vi "sta_Correlation Coefficient(SubVI).vi"(8 "에러 입력(에러 없음)":errorcluster, 10 "y":dbl[](array[numeric]), 11 "x":dbl[](array[numeric])) -> (0 "에러 출력":errorcluster, 1 "r^2":dbl format="%.7g", 2 "correlation coefficient r":dbl caption="상관 계수 r" format="%.7g", 3 "참조 번호 출력":refnum<k35>)   [LabVIEW 2018]
uses:
  PythonConfigGlobal.vi
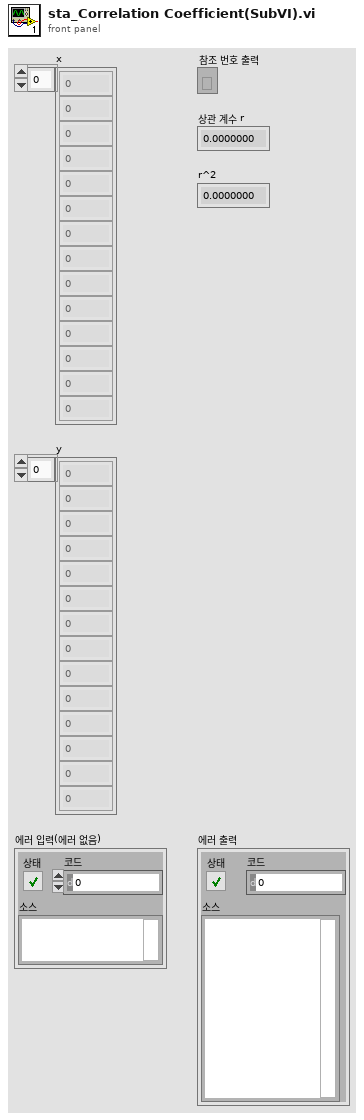
[diagram p1: front panel]
types:
  T1 = cluster{"session out":refnum<k35>, "appended path":path}
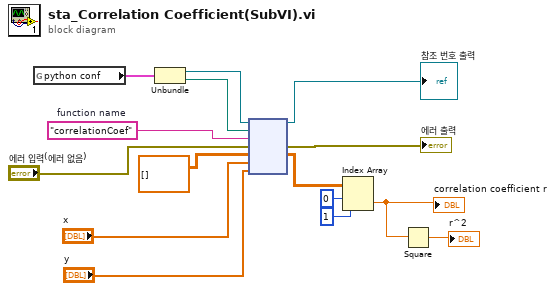
[diagram p0: block diagram]
diagram:
  w7 = "correlationCoef"  # function name
  n1 = global read "PythonConfigGlobal.vi" "python conf"() -> (w2:T1)
  n2 = Unbundle(w2) -> ("session out"=w6:refnum<k35>, "appended path"=w5:path)
  n3 = node(w6, w5, w7, "에러 입력(에러 없음)", dbl[][] [] ("x 2"), "x", "y") -> (→"참조 번호 출력":refnum<k35>, →"에러 출력":errorcluster, w11:dbl[][])  [unwired: 2 in, 2 out]
  n4 = Index Array(array=w11, index (row)=0 ("인덱스 (행)"), index (col)=1 ("비활성화된 인덱스 (열)")) -> (element=w14:dbl)
  "correlation coefficient r" <- w14
  n5 = Square(x=w14) -> (x^2=→"r^2":dbl)
